vi "Read When.vi"(8 "error in (no error)":errorcluster, 11 "TTLController in":refnum<class "TTLController.lvclass">) -> (0 "error out":errorcluster, 2 "String":string, 3 "TTLController out":refnum<class "TTLController.lvclass">)   [LabVIEW 2020, in "TTLController.lvclass"]
uses:
  TTLController.lvclass
  TTLController.lvclass/TTLController.ctl
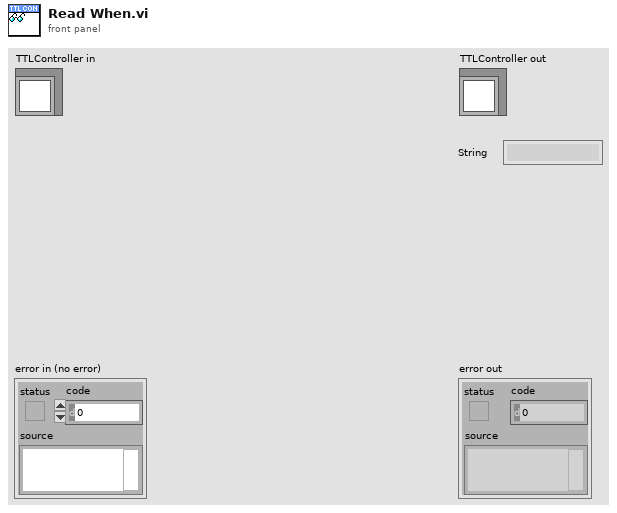
[diagram p1: front panel]
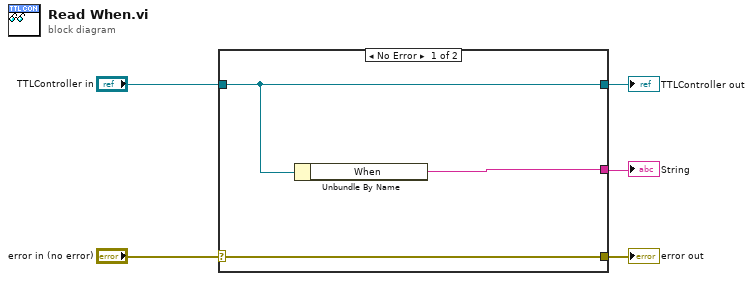
[diagram p0: block diagram]
diagram:
  n1 = case shown="No Error" "error in (no error)" {
    selector: "error in (no error)" -> [w8 w9]
    tunnel: [w8 w9] -> w4
    tunnel: [w7 w10] -> w2
    tunnel: "TTLController in" -> [w7 w10]
    tunnel: [w6 _] -> w1
    frame No Error {
      n2 = Unbundle By Name(w7) -> ("When"=w6:string)
    }
    frame Error {
    }
  }
  "error out" <- w4
  "TTLController out" <- w2
  "String" <- w1
